vi "deinitializeProgram.vi"   [LabVIEW 2015]
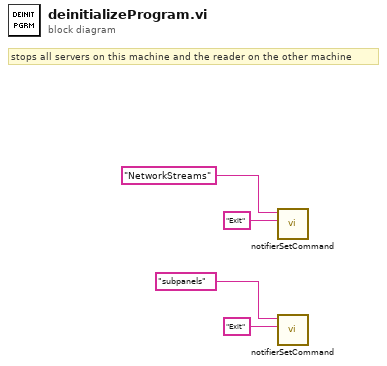
[diagram p0: block diagram]
diagram:
  # "stops all servers on this machine and the reader on the other machine"
  n1 = call "notifierSetCommand.vi"("set command"="Exit", "notifier listener name"="NetworkStreams") -> ()  [unwired: 9 in, 1 out]
  n2 = call "notifierSetCommand.vi"("set command"="Exit", "notifier listener name"="subpanels") -> ()  [unwired: 9 in, 1 out]
